vi "Set Framed Test Channel Path.vi"(8 "error in (no error)":errorcluster, 10 "Framed Test Channel Path":path, 11 "Test Channel Model in":refnum<class "Test Channel Model.lvclass">) -> (0 "error out":errorcluster, 3 "Test Channel Model out":refnum<class "Test Channel Model.lvclass">)   [LabVIEW 2013, in "Test Channel Model.lvlib" / "Test Channel Model.lvclass"]
uses:
  Test Channel Model.lvclass
  Test Channel Model.lvclass/Test Channel Model.ctl
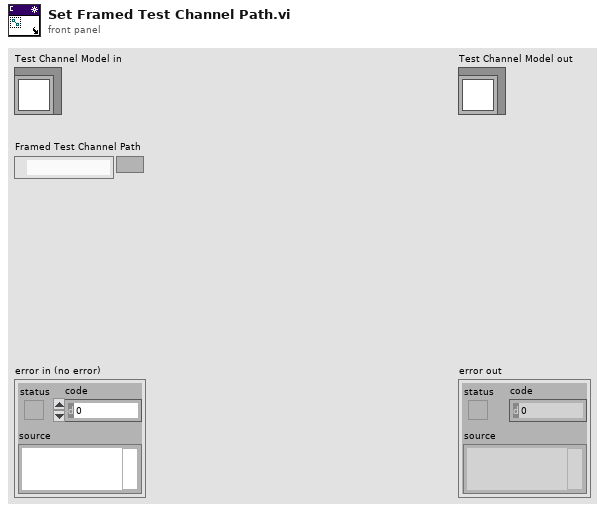
[diagram p1: front panel]
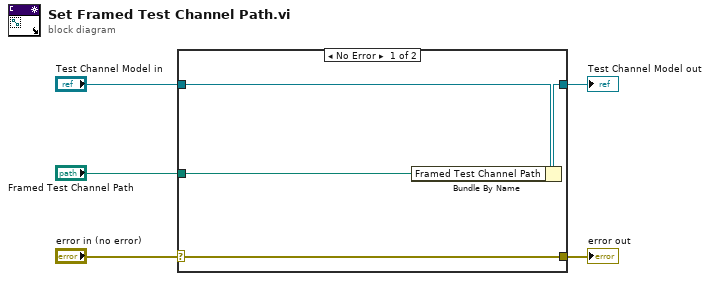
[diagram p0: block diagram]
diagram:
  n1 = case shown="No Error" "error in (no error)" {
    selector: "error in (no error)" -> [w9 w10]
    tunnel: [w9 w10] -> w4
    tunnel: [w7 w11] -> w2
    tunnel: "Test Channel Model in" -> [w8 w11]
    tunnel: "Framed Test Channel Path" -> [w6 _]
    frame No Error {
      n2 = Bundle By Name(cluster=w8, "Framed Test Channel Path"=w6) -> (w7:refnum<class "Test Channel Model.lvclass">)
    }
    frame Error {
    }
  }
  "error out" <- w4
  "Test Channel Model out" <- w2
